vi "Sentuator_US331-000005-100PA.vi"(6 "Atm Offset":dbl, 8 "error in (no error)":errorcluster, 10 "Density of Water":dbl, 11 "Depth sensor \nVoltage":dbl) -> (0 "error out 2":errorcluster, 2 "PSI":dbl(knob), 3 "Actual Depth (m)":dbl(slide))   [LabVIEW 2012]
panel:
  out "Raw Voltage":dbl(graph)
  out "PSI":dbl(graph)
  out "Absolute Depth (m)":dbl(slide)
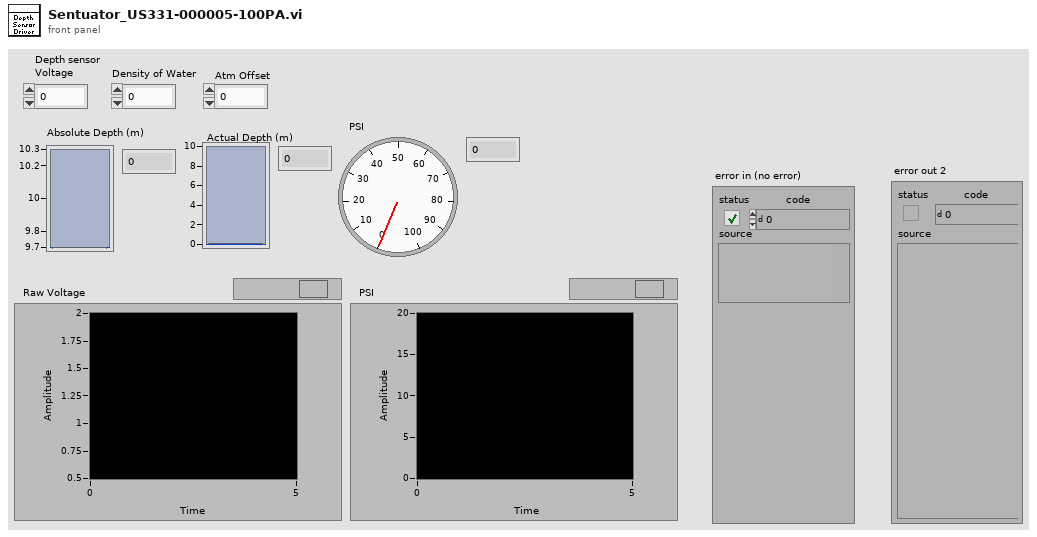
[diagram p1: front panel]
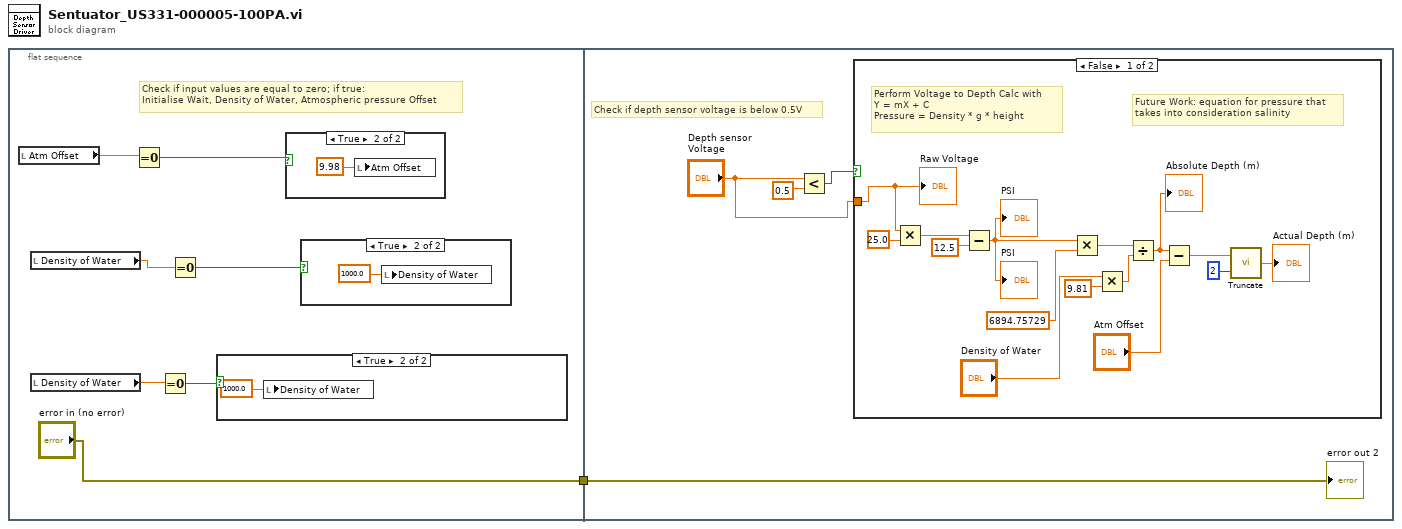
[diagram p0: block diagram]
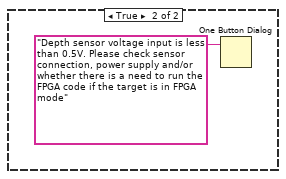
[diagram p5: hidden frame]
diagram:
  n1 = flat-sequence {
    tunnel: ["error in (no error)"] -> w1
    tunnel: w1 -> [w15]
    frame #0 {
      # "Check if input values are equal to zero; if true: \nInitialise Wait, Density of Water, Atmospheric pressure Offset"
      n2 = local read "Atm Offset"() -> (w8:dbl)
      n3 = local read "Density of Water"() -> (w6:dbl)
      n4 = local read "Density of Water"() -> (w4:dbl)
      n5 = Equal To 0?(x=w8) -> (x = 0?=w7:bool)
      n6 = Equal To 0?(x=w4) -> (x = 0?=w3:bool)
      n7 = Equal To 0?(x=w6) -> (x = 0?=w5:bool)
      n8 = case shown="True" w3 {
        frame False {
        }
        frame True {
          n9 = local write "Density of Water"(1000.0) -> ()
        }
      }
      n10 = case shown="True" w7 {
        frame False {
        }
        frame True {
          n11 = local write "Atm Offset"(9.98) -> ()
        }
      }
      n12 = case shown="True" w5 {
        frame False {
        }
        frame True {
          n13 = local write "Density of Water"(1000.0) -> ()
        }
      }
    }
    frame #1 {
      # "Check if depth sensor voltage is below 0.5V"
      n14 = Less?(x="Depth sensor \nVoltage", y=0.5) -> (x < y?=w14:bool)
      n15 = case shown="False" w14 {
        tunnel: "Depth sensor \nVoltage" -> [w16 _]
        frame False {
          # "Future Work: equation for pressure that\ntakes into consideration salinity"
          # "Perform Voltage to Depth Calc with\nY = mX + C\nPressure = Density * g * height"
          n16 = Multiply(x=w16, y=25.0) -> (x*y=w29:dbl)
          n17 = Subtract(x=w29, y=12.5) -> (x-y=w22:dbl)
          "PSI" <- w22
          "PSI" <- w22
          n18 = Multiply(x=w22, y=6894.75729) -> (x*y=w21:dbl)
          n19 = Multiply(x="Density of Water", y=9.81) -> (x*y=w25:dbl)
          n20 = Divide(x=w21, y=w25) -> (x/y=w20:dbl)
          "Absolute Depth (m)" <- w20
          n21 = Subtract(x=w20, y="Atm Offset") -> (x-y=w19:dbl)
          n22 = call "Truncate.vi"("Number of Digits"=i16 2, "Number"=w19) -> ("Truncated Number"=→"Actual Depth (m)":dbl)
          "Raw Voltage" <- w16
        }
        frame True {
          n23 = One Button Dialog(message="Depth sensor voltage input is less than 0.5V. Please check sensor connection, power supply and/or whether there is a need to run the FPGA code if the target is in FPGA mode") -> ()  [unwired: 1 in, 1 out]
        }
      }
      "error out 2" <- w15
    }
  }
